vi "host.vi"() -> ()   [LabVIEW 2020]
uses:
  b4957acc-33c7-4f51-b6c8-be02e890b770.vi
  <vilib>/Array/Sort 2D Array - Pop Stack.vi
  <vilib>/Array/Sort 2D Array - Push Stack.vi
  b4957acc-33c7-4f51-b6c8-be02e890b770.vi/269d4b3b-47f5-49e3-8884-44851e4dd9d5.vi
  b4957acc-33c7-4f51-b6c8-be02e890b770.vi/6d99389c-673d-4efb-bf33-19b32bcf4cf8.vi
  <vilib>/FPGAPlugInAG/cRIO-9035/niLvFpga_Open_cRIO-9035.vi
  <vilib>/FPGAPlugInAG/cRIO-9035/niLvFpga_Reset_cRIO-9035.vi
  <vilib>/Utility/error.llb/Error Cluster From Error Code.vi
  <vilib>/rvi/errors/niLvFpgaAdjustHostInterfaceError.vi
  <vilib>/FPGAPlugInAG/cRIO-9035/niLvFpga_Run_cRIO-9035.vi
  <vilib>/FPGAPlugInAG/cRIO-9035/niLvFpga_Close_cRIO-9035.vi
  <vilib>/rvi/interface/nirviOpenFPGA/nirviOpenFPGA.xnode
  FPGA Bitfiles/project_FPGATarget_target_HTaLvjA4zSY.lvbitx
  target.vi
  <vilib>/rvi/interface/nirviMethod/nirviMethod.xnode
  <vilib>/rvi/interface/nirviReadWriteControl/nirviReadWriteControl.xnode
  <vilib>/rvi/interface/nirviCloseFPGA/nirviCloseFPGA.xnode
  <vilib>/Analysis/NI_AALBase.lvlib
  <vilib>/FPGAPlugInAG/cRIO-9035/niLvFpga_StartFifo_cRIO-9035.vi
  <vilib>/rvi/errors/niLvFpgaMergeErrorWithErrorCode.vi
  <vilib>/FPGAPlugInAG/cRIO-9035/niLvFpga_WriteFifo_cRIO-9035.vi
  <vilib>/FPGAPlugInAG/cRIO-9035/niLvFpga_ReadFifo_cRIO-9035.vi
  NiFpgaLv.dll
panel:
  out "error out":errorcluster
  out "Timed Out? FIFO out index":bool
  out "Timed Out? FIFO out IMG":bool
  out "Timed Out? FIFO out REAL":bool
  out "Timed Out? FIFO in REAL":bool
  out "Timed Out? FIFO in IMG":bool
  out "sorted signal 3":dbl[](graph)
  out "Data":fxp<+/-,32,21>[](array[numeric])
  out "sorted signal 2":dbl[](graph)
  out "index values":i32[](array[numeric])
  out "sorted 2D array":dbl[][](array[numeric])
  out "appended array":dbl[][](array[numeric])
  out "sorted array":dbl[](array[numeric])
  out "uniform white noise":dbl[](array[numeric])
  out "Waveform Graph":sgl[](graph)
  out "sort time (ms)":dbl
  out "Elements Remaining":u32
  out "sorted signal":dbl[](graph)
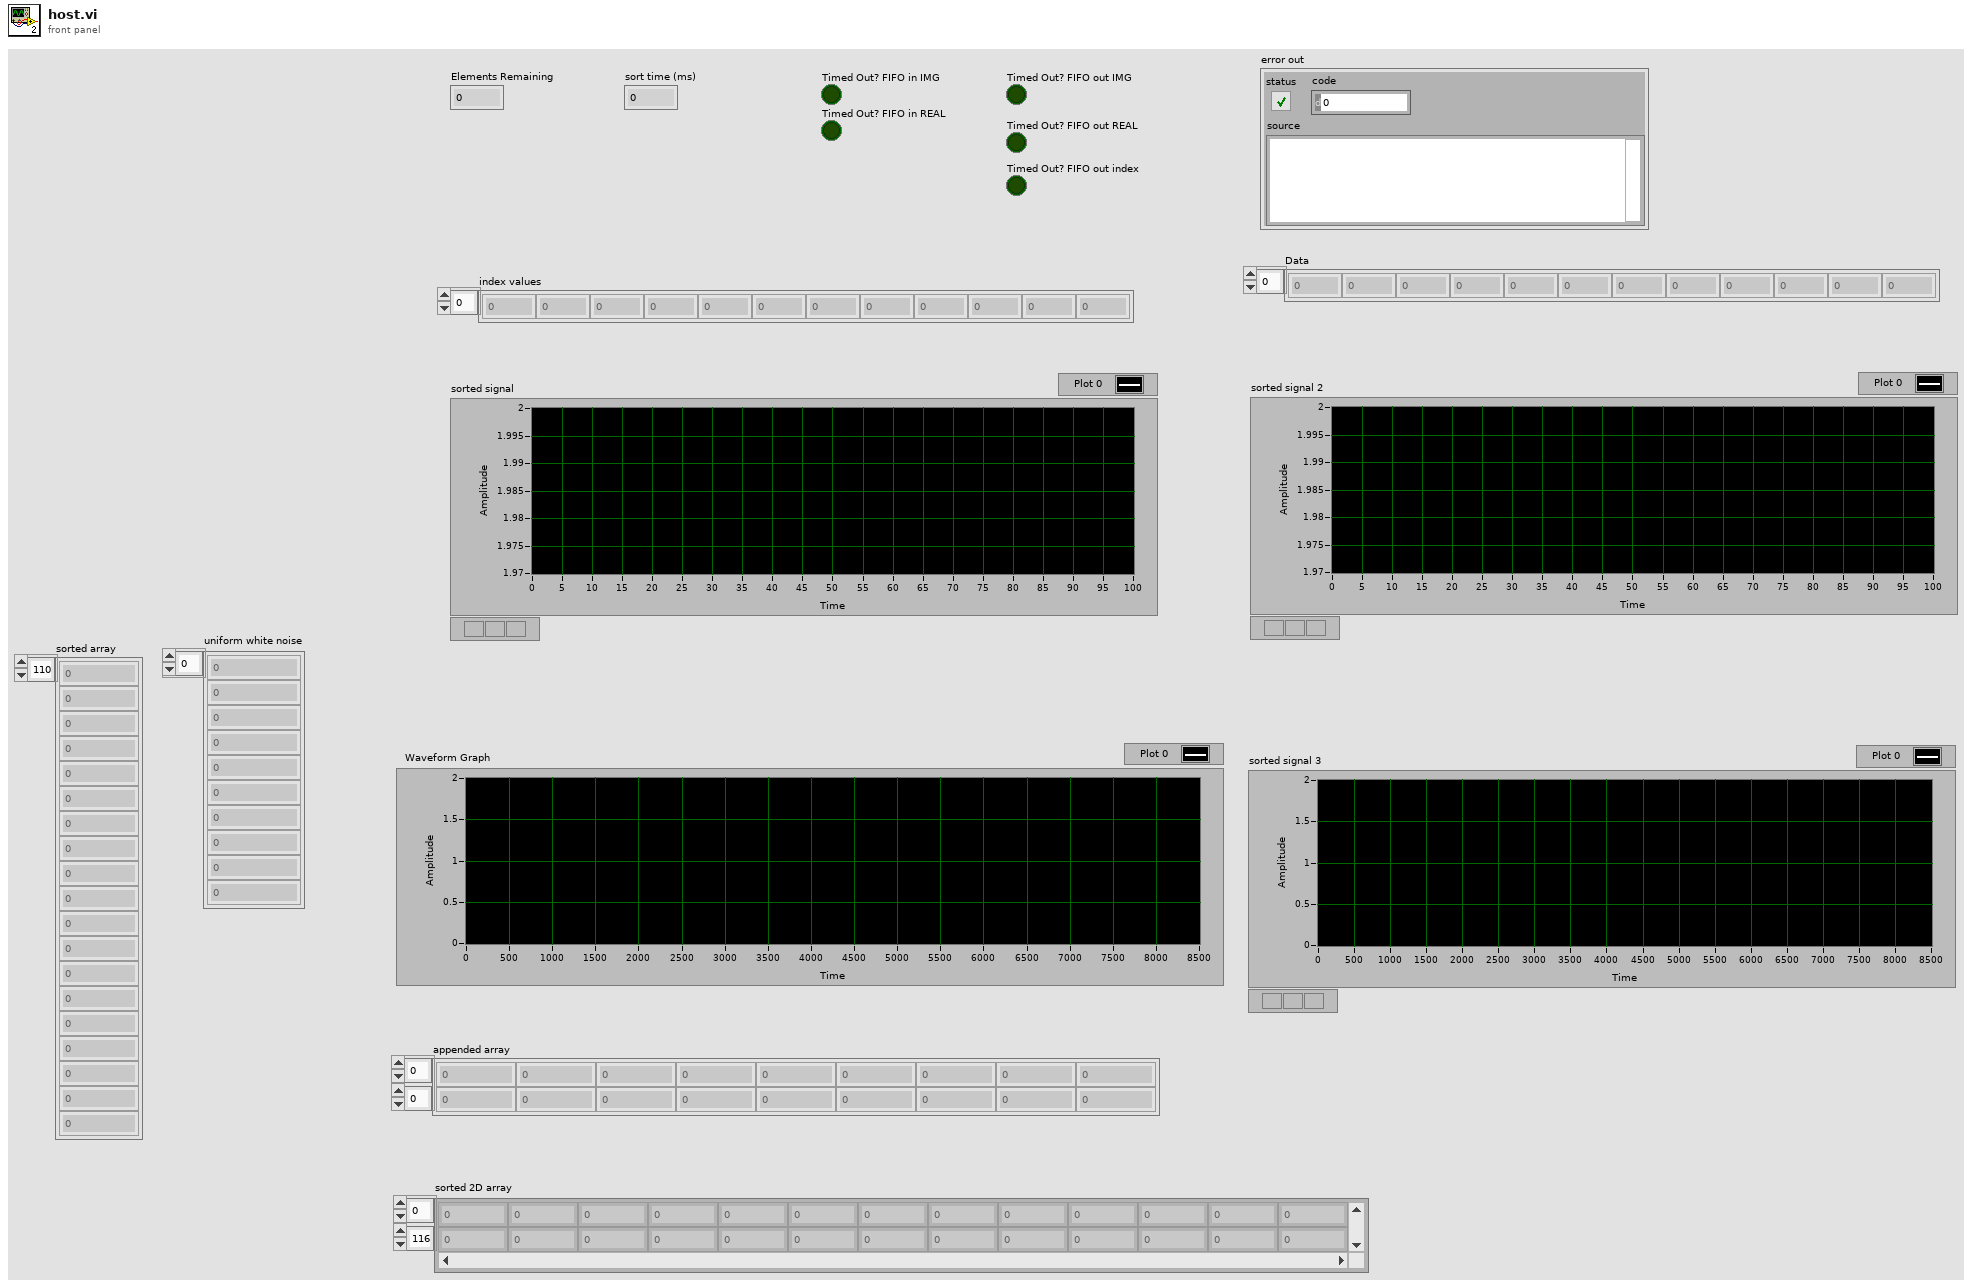
[diagram p1: front panel]
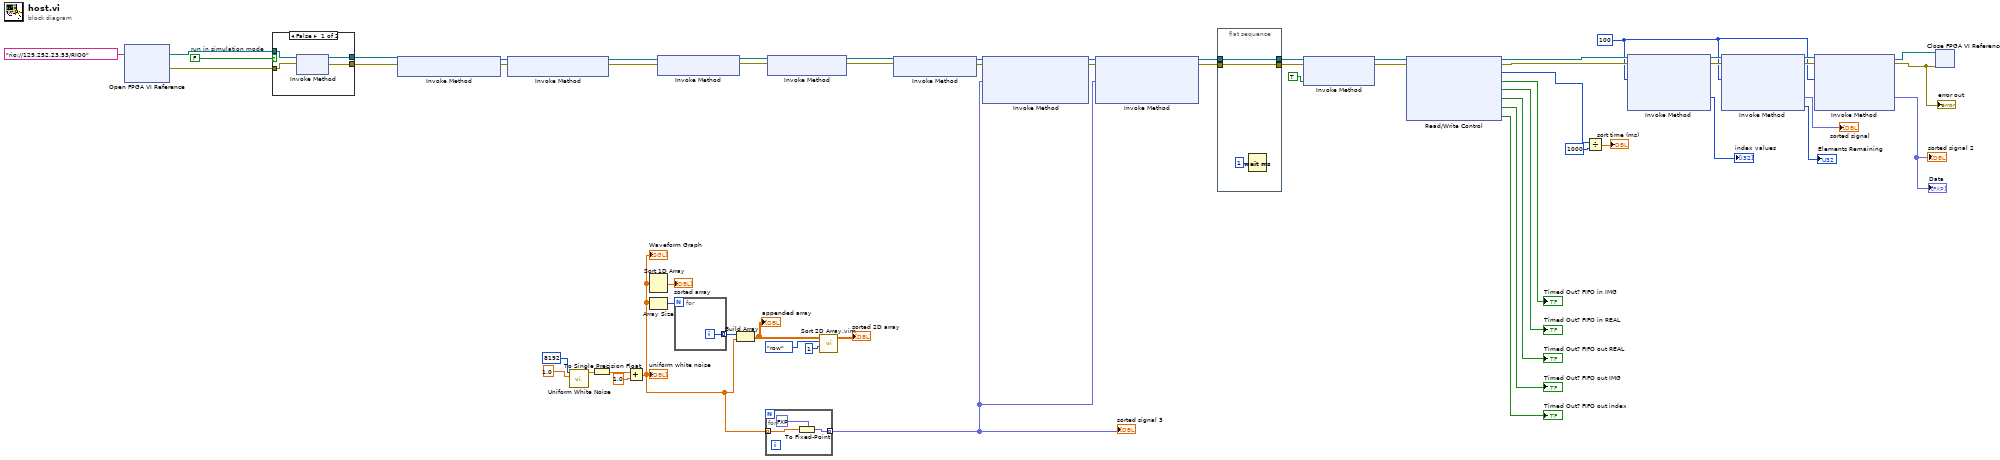
[diagram p0: block diagram]
diagram:
  w5 = FALSE  # run in simulation mode
  w23 = u32 100 ("Number of Elements")
  n1 = xnode "Open FPGA VI Reference"("resource name"=tag "rio://129.252.23.53/RIO0") -> ("FPGA VI Reference Out"=w4:refnum<k20>, "error out"=w3:errorcluster)  [unwired: 1 in]
  n2 = case shown="False" w5 {
    tunnel: w4 -> [w64 w65]
    tunnel: w3 -> [w63 w66]
    tunnel: [w62 w65] -> w2
    tunnel: [w61 w66] -> w1
    frame False {
      n3 = xnode "Invoke Method"("FPGA VI Reference In"=w64, "error in"=w63) -> ("FPGA VI Reference Out"=w62:refnum<k20>, "error out"=w61:errorcluster)
    }
    frame True {
    }
  }
  n4 = xnode "Invoke Method"("FPGA VI Reference In"=w2, "error in"=w1) -> ("FPGA VI Reference Out"=w33:refnum<k20>, "error out"=w32:errorcluster)
  n5 = xnode "Invoke Method"("FPGA VI Reference In"=w33, "error in"=w32) -> ("FPGA VI Reference Out"=w18:refnum<k20>, "error out"=w17:errorcluster)
  n6 = call <vilib>:"Uniform White Noise.vi"("amplitude"=1.0, "samples"=8192) -> ("uniform white noise"=w36:dbl[])  [unwired: 8 in, 1 out]
  n7 = To Single Precision Float(number=w36) -> (single precision float=w35:sgl[])
  n8 = Add(x=w35, y=sgl 1.0 ("amplitude")) -> (x+y=w34:sgl[])
  "Waveform Graph" <- w34
  "uniform white noise" <- w34
  n9 = Sort 1D Array(array=w34) -> (sorted array=→"sorted array":sgl[])
  n10 = Array Size(array=w34) -> (size(s)=w43:i32)
  n11 = xnode "Invoke Method"("FPGA VI Reference In"=w18, "error in"=w17) -> ("FPGA VI Reference Out"=w16:refnum<k20>, "error out"=w21:errorcluster)
  n12 = for {
    N: w43 -> [_]
    tunnel: [w67] -> w42 mode=indexing
    i -> [w67]
  }
  n13 = Build Array(w42, w34) -> (w41:sgl[][])
  "appended array" <- w41
  n14 = for {
    tunnel: w34 -> [w70] mode=indexing
    tunnel: [w69] -> w15 mode=indexing
    n15 = To Fixed-Point(fixed-point type=fxp<+/-,32,21> 0.0, number=w70) -> (fixed-point=w69:fxp<+/-,32,21>)
  }
  "sorted signal 3" <- w15
  n16 = xnode "Invoke Method"("FPGA VI Reference In"=w16, "error in"=w21) -> ("FPGA VI Reference Out"=w20:refnum<k20>, "error out"=w19:errorcluster)
  n17 = call "Sort 2D Array.vim"("index"=1, "dimension to index (column)"=enum16{"column", "row"}."row", "2D array"=w41) -> ("sorted 2D array"=→"sorted 2D array":sgl[][])  [unwired: 7 in, 1 out]
  n18 = xnode "Invoke Method"("FPGA VI Reference In"=w20, "error in"=w19) -> ("FPGA VI Reference Out"=w31:refnum<k20>, "error out"=w30:errorcluster)
  n19 = xnode "Invoke Method"("FPGA VI Reference In"=w31, "error in"=w30, "Data"=w15) -> ("FPGA VI Reference Out"=w29:refnum<k20>, "error out"=w28:errorcluster)  [unwired: 1 in, 1 out]
  n20 = xnode "Invoke Method"("FPGA VI Reference In"=w29, "error in"=w28, "Data"=w15) -> ("FPGA VI Reference Out"=w8:refnum<k20>, "error out"=w6:errorcluster)  [unwired: 1 in, 1 out]
  n21 = flat-sequence {
    tunnel: [w72] -> w9
    tunnel: w8 -> [w72]
    tunnel: [w71] -> w7
    tunnel: w6 -> [w71]
    frame #0 {
      n22 = Wait (ms)(milliseconds to wait=u32 1) -> ()  [unwired: 1 out]
    }
  }
  n23 = xnode "Invoke Method"("FPGA VI Reference In"=w9, "error in"=w7, "Wait Until Done (F)"=TRUE) -> ("FPGA VI Reference Out"=w57:refnum<k20>, "error out"=w56:errorcluster)
  n24 = xnode "Read/Write Control"("FPGA VI Reference In"=w57, "error in"=w56) -> ("FPGA VI Reference Out"=w51:refnum<k20>, "error out"=w49:errorcluster, "sort time (us)"=w55:u32, "Timed Out? FIFO in IMG"=→"Timed Out? FIFO in IMG":bool, "Timed Out? FIFO in REAL"=→"Timed Out? FIFO in REAL":bool, "Timed Out? FIFO out REAL"=→"Timed Out? FIFO out REAL":bool, "Timed Out? FIFO out IMG"=→"Timed Out? FIFO out IMG":bool, "Timed Out? FIFO out index"=→"Timed Out? FIFO out index":bool)
  n25 = Divide(x=w55, y=u32 1000) -> (x/y=→"sort time (ms)":dbl)
  n26 = xnode "Invoke Method"("FPGA VI Reference In"=w51, "error in"=w49, "Number of Elements"=w23) -> ("FPGA VI Reference Out"=w50:refnum<k20>, "error out"=w48:errorcluster, "Data"=→"index values":i32[])  [unwired: 1 in, 1 out]
  n27 = xnode "Invoke Method"("FPGA VI Reference In"=w50, "error in"=w48, "Number of Elements"=w23) -> ("FPGA VI Reference Out"=w27:refnum<k20>, "error out"=w26:errorcluster, "Data"=→"sorted signal":fxp<+/-,32,21>[], "Elements Remaining"=→"Elements Remaining":u32)  [unwired: 1 in]
  n28 = xnode "Invoke Method"("FPGA VI Reference In"=w27, "error in"=w26, "Number of Elements"=w23) -> ("FPGA VI Reference Out"=w25:refnum<k20>, "error out"=w24:errorcluster, "Data"=→"sorted signal 2" →"Data":fxp<+/-,32,21>[])  [unwired: 1 in, 1 out]
  "error out" <- w24
  n29 = xnode "Close FPGA VI Reference"("FPGA VI Reference In"=w25, "error in"=w24) -> ()  [unwired: 1 out]
